vi "Reports.Result Report Config, Read or Write.vi"(8 "error in (no error)":errorcluster, 9 "Read(F)/Write(T)":bool, 10 "Report Config In":T1[](array[typedef]), 11 "Config Folder":path) -> (0 "error out":errorcluster, 2 "Report Config Out":T1[](array[typedef]))   [LabVIEW 2024]
uses:
  Report.Result Report Config.ctl
  Report.Result Report File Type.ctl
  <vilib>/KATE/Files/File Utils.lvlib
panel:
  out "JSON string":string
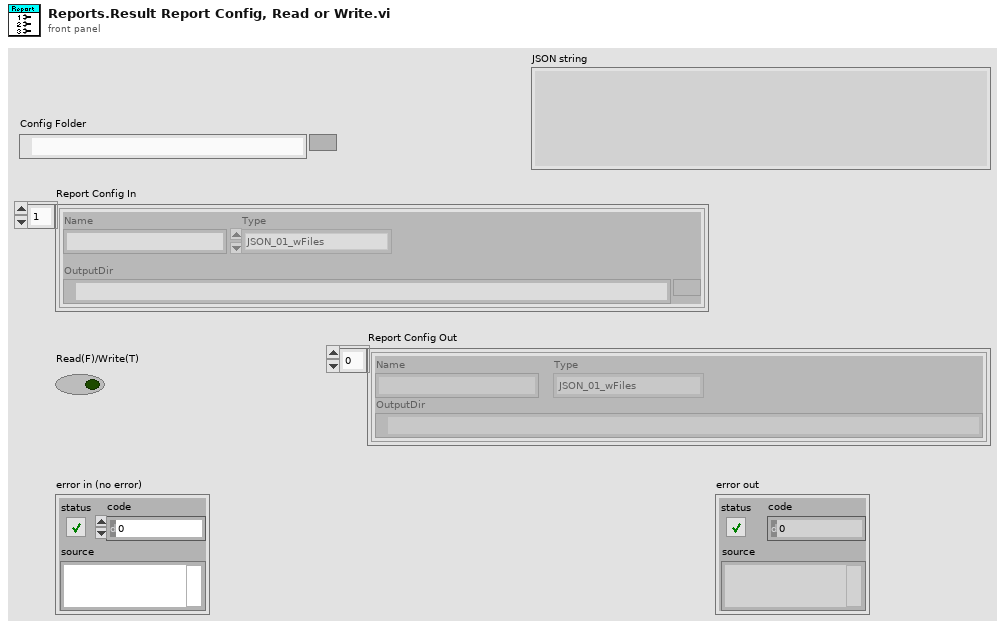
[diagram p1: front panel]
types:
  T1 = typedef "Report.Result Report Config.ctl" = cluster{"Name":string, "Type":T2, "OutputDir":path}
  T2 = typedef "Report.Result Report File Type.ctl" = enum16{"Xlink", "XML_01", "XML_01_wFiles", "JSON_01", "JSON_01_wFiles"}
  T3 = cluster{"Name":string, "Type":string, "Path":string}
  T4 = cluster{"Reports":cluster{"Name":string, "Type":string, "Path":string}[]}
  T5 = cluster{"Name":string, "Type":string, "Path":string}[]
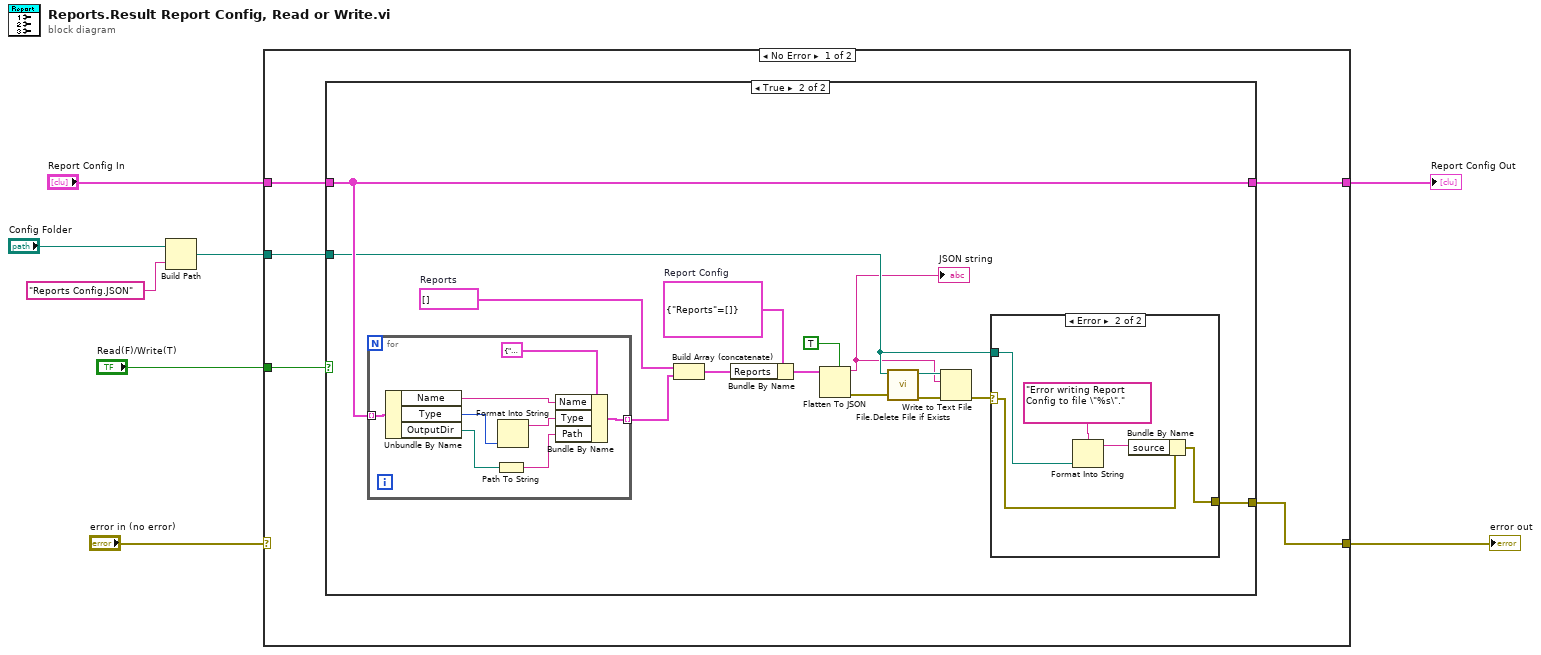
[diagram p0: block diagram]
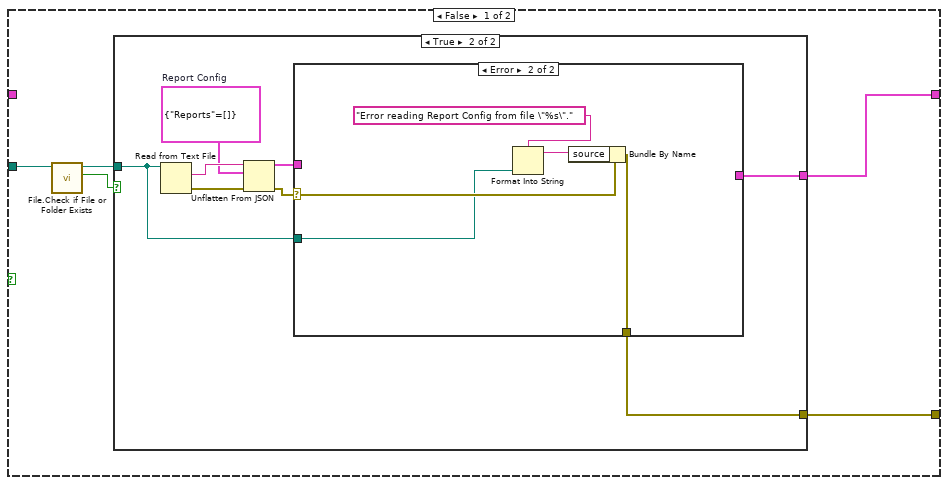
[diagram p2: hidden frame]
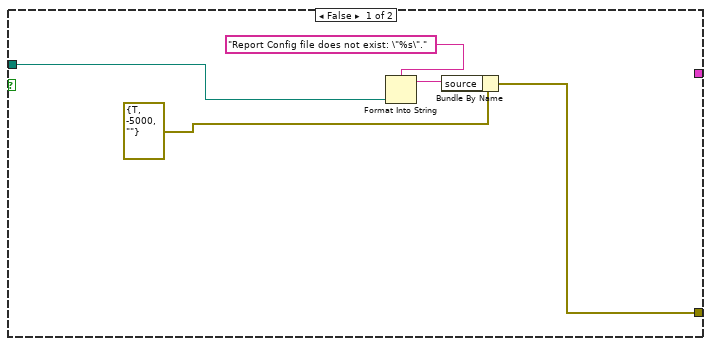
[diagram p3: hidden frame]
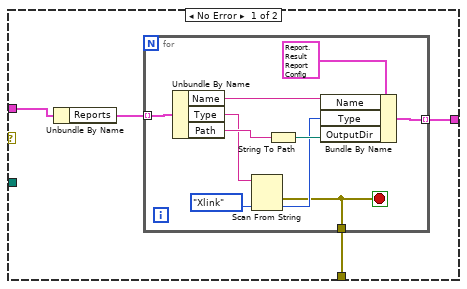
[diagram p4: hidden frame]
diagram:
  n1 = Build Path(base path="Config Folder", name or relative path="Reports Config.JSON") -> (appended path=w2:path)
  n2 = case shown="No Error" "error in (no error)" {
    selector: "error in (no error)" -> [_ w78]
    tunnel: "Read(F)/Write(T)" -> [w13 _]
    tunnel: "Report Config In" -> [w12 w79]
    tunnel: [w9 w79] -> w1
    tunnel: [w10 w78] -> w3
    tunnel: w2 -> [w11 _]
    frame No Error {
      n3 = case shown="True" w13 {
        tunnel: w12 -> [_ w62]
        tunnel: w11 -> [w16 w55]
        tunnel: [w17 w56] -> w10
        tunnel: [w18 w62] -> w9
        frame False {
          n4 = call <vilib>:"File.Check if File or Folder Exists.vi"("Path"=w16) -> ("Exists"=w14:bool, "Dup Path"=w15:path)  [unwired: 6 in, 3 out]
          n5 = case shown="True" w14 {
            tunnel: [_ w29] -> w18
            tunnel: [w19 w28] -> w17
            tunnel: w15 -> [w20 w24]
            frame False {
              n6 = Format Into String(format string="Report Config file does not exist: \"%s\".", w20) -> (resulting string=w23:string)  [unwired: 2 in, 1 out]
              n7 = Bundle By Name(cluster=errorcluster {"status"=TRUE, "code"=-5000, "source"=""} ("error constant"), "source"=w23) -> (w19:errorcluster)
            }
            frame True {
              w25 = T4 {"Reports"=[]}  # Report Config
              n8 = Read from Text File(file (use dialog)=w24) -> (text=w31:string, error out=w26:errorcluster)  [unwired: 3 in, 2 out]
              n9 = Unflatten From JSON(JSON string=w31, type and defaults=w25, error in (no error)=w26) -> (value=w30:T4, error out=w27:errorcluster)  [unwired: 4 in]
              n10 = case shown="Error" w27 {
                selector: w27 -> [_ w50]
                tunnel: w30 -> [w33 _]
                tunnel: [w35 _] -> w29
                tunnel: [w34 w49] -> w28
                tunnel: w24 -> [_ w46]
                frame No Error {
                  n11 = Unbundle By Name(w33) -> ("Reports"=w32:T5)
                  n12 = for {
                    tunnel: w32 -> [w45] mode=indexing
                    tunnel: [w41] -> w35 mode=indexing
                    tunnel: [w36] -> w34
                    stop <- w36 stop-if-true
                    n13 = Unbundle By Name(w45) -> ("Name"=w43:string, "Type"=w39:string, "Path"=w44:string)
                    n14 = Scan From String(input string=w39, default 1=Report.Result_Report_File_Type."Xlink" ("Type")) -> (error out=w36:errorcluster, output 1=w37:T2)  [unwired: 3 in, 2 out]
                    n15 = String To Path(string=w44) -> (path=w42:path)
                    n16 = Bundle By Name(cluster=T1 {"Name"="", "Type"=enum."JSON_01_wFiles", "OutputDir"=path ""} ("Report Config In"), "Name"=w43, "Type"=w37, "OutputDir"=w42) -> (w41:T1)
                  }
                }
                frame Error {
                  n17 = Format Into String(format string="Error reading Report Config from file \"%s\".", w46) -> (resulting string=w48:string)  [unwired: 2 in, 1 out]
                  n18 = Bundle By Name(cluster=w50, "source"=w48) -> (w49:errorcluster)
                }
              }
            }
          }
        }
        frame True {
          w59 = T4 {"Reports"=[]}  # Report Config
          w60 = T5 []  # Reports
          n19 = for {
            tunnel: w62 -> [w77] mode=indexing
            tunnel: [w70] -> w61 mode=indexing
            n20 = Unbundle By Name(w77) -> ("Name"=w73:string, "Type"=w76:T2, "OutputDir"=w75:path)
            n21 = Path To String(path=w75) -> (string=w71:string)
            n22 = Format Into String(w76) -> (resulting string=w72:string)  [unwired: 3 in, 1 out]
            n23 = Bundle By Name(cluster=T3 {"Name"="", "Type"="", "Path"=""} ("Report"), "Name"=w73, "Type"=w72, "Path"=w71) -> (w70:T3)
          }
          n24 = Build Array (concatenate)(w60, w61) -> (w58:T5)
          n25 = Bundle By Name(cluster=w59, "Reports"=w58) -> (w57:T4)
          n26 = Flatten To JSON(enable LabVIEW extensions? (T)=TRUE, anything=w57) -> (JSON string=w51:string, 11:w63:errorcluster)  [unwired: 1 in]
          "JSON string" <- w51
          n27 = call "File.Delete File if Exists.vi"("error in"=w63, "Path"=w55) -> ("error out"=w54:errorcluster, "Path Out"=w53:path)  [unwired: 8 in]
          n28 = Write to Text File(file (use dialog)=w53, text=w51, error in=w54) -> (error out=w52:errorcluster)  [unwired: 1 in, 2 out]
          n29 = case shown="Error" w52 {
            selector: w52 -> [_ w67]
            tunnel: [_ w66] -> w56
            tunnel: w55 -> [_ w65]
            frame No Error {
            }
            frame Error {
              n30 = Format Into String(format string="Error writing Report Config to file \"%s\".", w65) -> (resulting string=w69:string)  [unwired: 2 in, 1 out]
              n31 = Bundle By Name(cluster=w67, "source"=w69) -> (w66:errorcluster)
            }
          }
        }
      }
    }
    frame Error {
    }
  }
  "error out" <- w3
  "Report Config Out" <- w1
